vi "Delimiter.vi"(8 "error in":errorcluster, 11 "Delimiter":string="localhost") -> (0 "error out":errorcluster, 3 "Delimiter":string)   [LabVIEW 2014]
doc: "<B>Copyrights</B>: (c) MHWirth 2015. All rights reserved.\n\nThis subVI sets the csv file delimeter."
panel:
  in  "Enum":T1(ring)
  in  "update":bool
  # "CSV Delimiter"
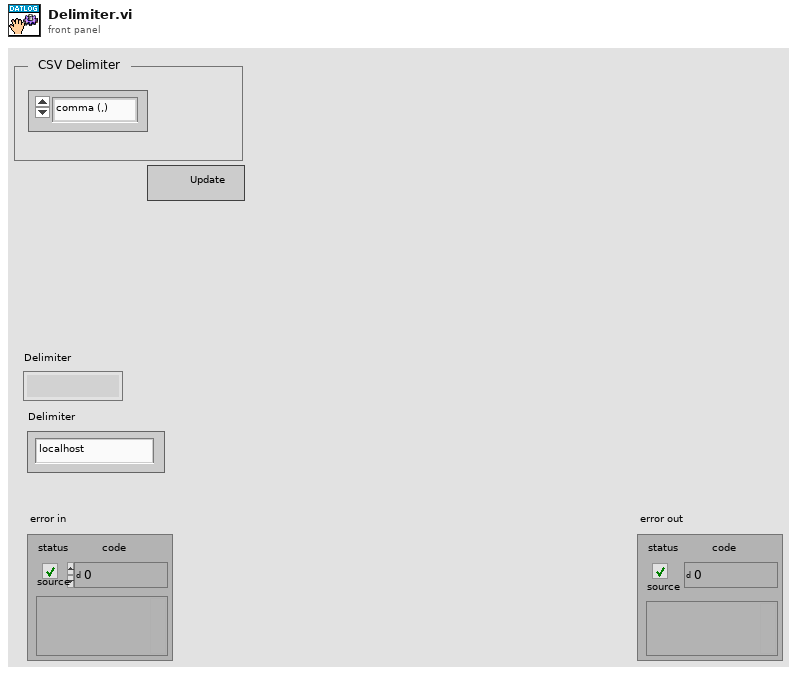
[diagram p1: front panel]
types:
  T1 = enum16{"comma (,)", "semi-colon (;)", "tab (/t)"}
  T2 = typedef "eventvkey.ctl" = enum16{"ASCII", "Enter", "Return", "Shift", "Ctrl", "Alt", "Cmd", "Opt", "Caps", "NumLock", "Clear", "Break", "Up", "Down", "Left", "Right", "Insert", "Delete", "Home", "End", "PageUp", "PageDown", "Escape", "Help", "Pause", "ScrollLock", "F1", "F2", "F3", "F4", "F5", "F6", "F7", "F8", "F9", "F10", "F11", "F12", "F13", "F14", "F15", "F16", "F17", "F18", "F19", "F20", "F21", "F22", "F23", "F24", "Play", "VolumeUp", "VolumeDown", "Mute", "Two Byte Char"}
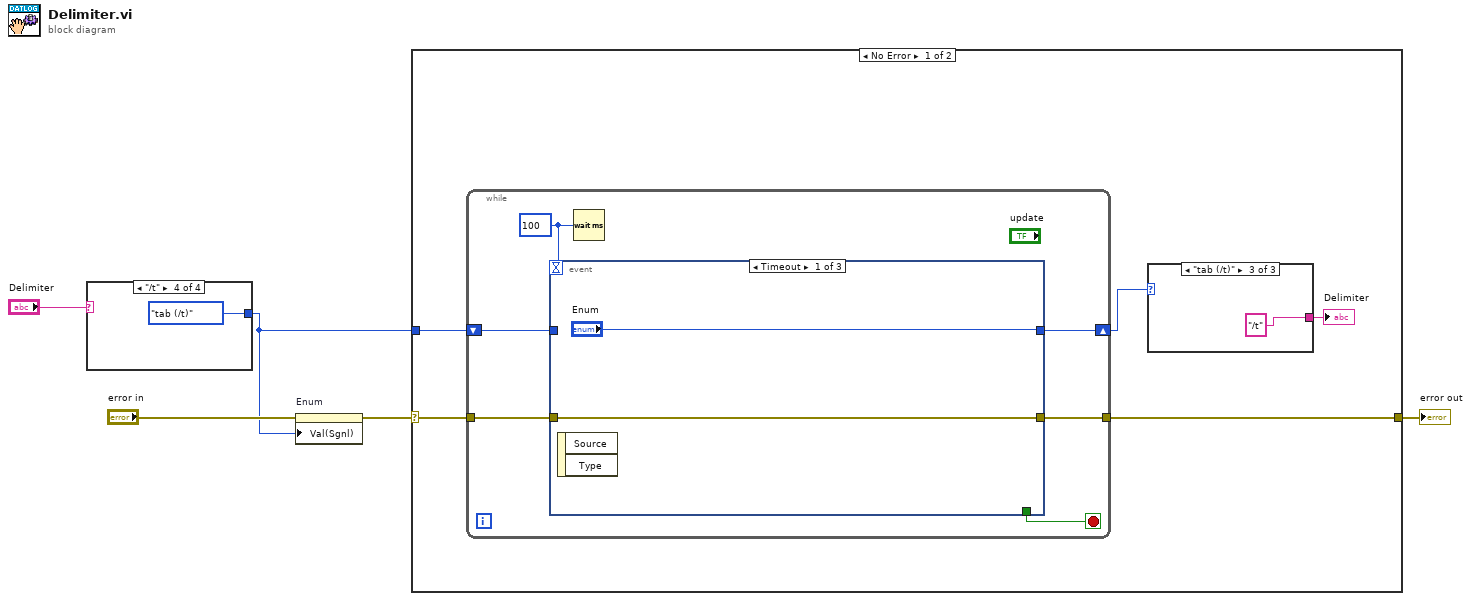
[diagram p0: block diagram]
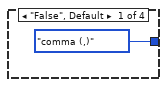
[diagram p2: hidden frame]
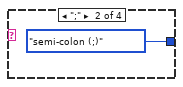
[diagram p3: hidden frame]
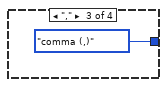
[diagram p4: hidden frame]
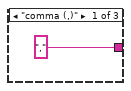
[diagram p5: hidden frame]
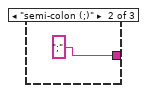
[diagram p6: hidden frame]
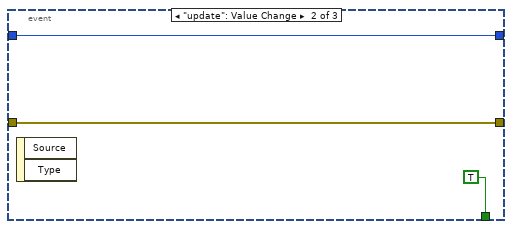
[diagram p7: hidden frame]
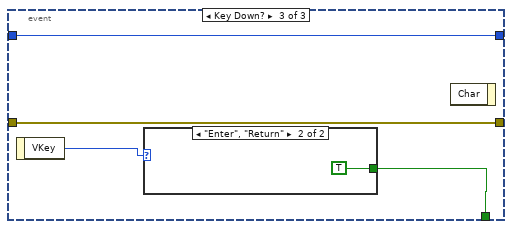
[diagram p8: hidden frame]
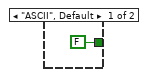
[diagram p9: hidden frame]
diagram:
  n1 = case shown="\"/t\"" "Delimiter" {
    tunnel: [T1."comma (,)" ("Enum") T1."semi-colon (;)" ("Enum") T1."comma (,)" ("Enum") T1."tab (/t)" ("Enum")] -> w1
    frame "False", Default {
    }
    frame ";" {
    }
    frame "," {
    }
    frame "/t" {
    }
  }
  n2 = property on="Enum" class="Enum (strict)"(error in="error in", "Val(Sgnl)"=w1) -> (error out=w2:errorcluster)  [unwired: 1 in, 1 out]
  n3 = case shown="No Error" w2 {
    selector: w2 -> [w14 w35]
    tunnel: [w13 w35] -> w5
    tunnel: w1 -> [w12 _]
    frame No Error {
      n4 = while {
        shift-right: [w21] -> w11
        shift-left: w12 -> [w23]
        tunnel: w14 -> [w19]
        tunnel: [w18] -> w13
        stop <- w20 stop-if-true
        w22 = u32 100 ("milliseconds to wait")
        n5 = event shown="[0] Timeout" {
          selector: _ -> [_ _ _]
          dyn-events: _ -> [_ _ _]
          timeout: w22 -> [_ _ _]
          tunnel: w23 -> [_ w27 w31]
          tunnel: ["Enum" w27 w31] -> w21
          tunnel: [_ TRUE w30] -> w20
          tunnel: w19 -> [w24 w26 w32]
          tunnel: [w24 w26 w32] -> w18
          event Timeout {
            n6 = event-data() -> ()  [unwired: 1 in, 2 out]
          }
          event "update": Value Change {
            n7 = event-data() -> ()  [unwired: 1 in, 2 out]
          }
          event Key Down? {
            n8 = event-data() -> ("VKey"=w29:T2)  [unwired: 1 in]
            n9 = case shown="\"Enter\", \"Return\"" w29 {
              tunnel: [FALSE TRUE] -> w30
              frame "ASCII", Default {
              }
              frame "Enter", "Return" {
              }
            }
            n10 = event-data() -> ()  [unwired: 2 in, 1 out]
          }
        }
        n11 = Wait (ms)(milliseconds to wait=w22) -> ()  [unwired: 1 out]
      }
      n12 = case shown="\"tab (/t)\"" w11 {
        tunnel: ["," ";" "/t"] -> w10
        frame "comma (,)" {
        }
        frame "semi-colon (;)" {
        }
        frame "tab (/t)" {
        }
      }
      "Delimiter" <- w10
    }
    frame Error {
    }
  }
  "error out" <- w5
